vi "2d_pose_estimation_euler_integral.vi"(4 "y_0":dbl, 6 "x_0":dbl, 7 "Zero XY?":bool, 9 "theta(rad)":dbl, 10 "v(per tick)":dbl) -> (1 "y":dbl, 2 "x":dbl)   [LabVIEW 2019]
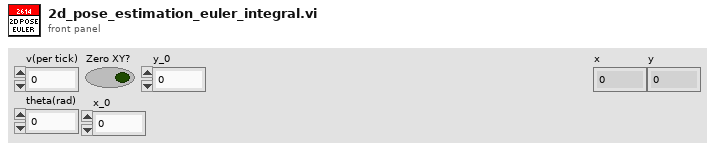
[diagram p1: front panel]
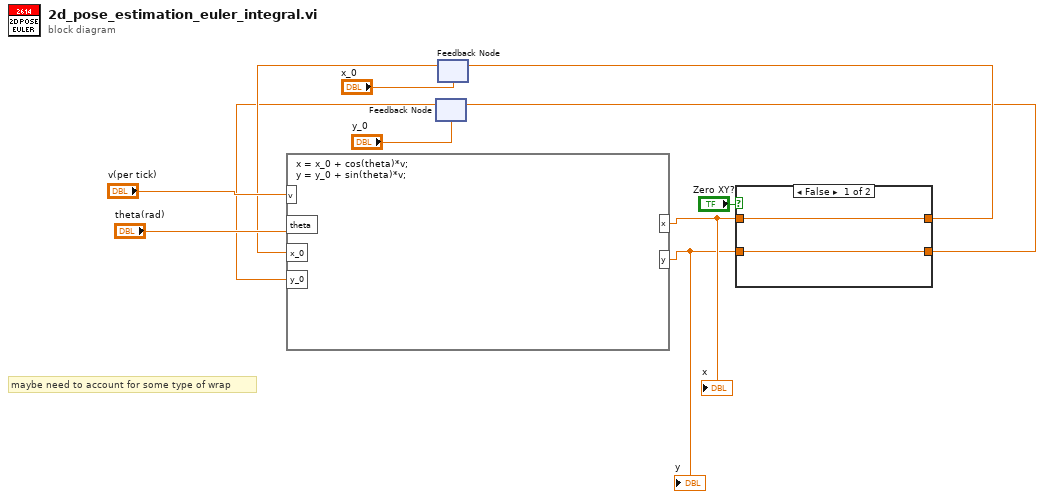
[diagram p0: block diagram]
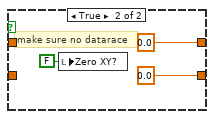
[diagram p2: hidden frame]
diagram:
  # "maybe need to account for some type of wrap"
  n1 = feedback #1("y_0") -> (w3:dbl)
  n2 = feedback #2("x_0") -> (w4:dbl)
  n3 = formula code="x = x_0 + cos(theta)*v;\ny = y_0 + sin(theta)*v;"("v"="v(per tick)", "theta"="theta(rad)", "x_0"=w4, "y_0"=w3) -> ("x"=w6:dbl, "y"=w5:dbl)
  "x" <- w6
  "y" <- w5
  n4 = case shown="False" "Zero XY?" {
    tunnel: [w13 0.0 ("output variable")] -> w8
    tunnel: [w12 0.0 ("output variable")] -> w7
    tunnel: w6 -> [w13 _]
    tunnel: w5 -> [w12 _]
    frame False {
    }
    frame True {
      # "make sure no datarace"
      n5 = local write "Zero XY?"(FALSE ("Zero XY?")) -> ()
    }
  }
  n6 = feedback-in #1(w7) -> ()
  n7 = feedback-in #2(w8) -> ()
